vi "Program Set Point.vi"(8 "error in (no error)":errorcluster, 10 "Set Point":dbl, 11 "LakeShore T Controller in":refnum<class "LakeShore T Controller.lvclass">) -> (0 "error out":errorcluster, 3 "LakeShore T Controller out":refnum<class "LakeShore T Controller.lvclass">)   [LabVIEW 2015, in "LakeShore T Controller.lvclass"]
uses:
  LakeShore T Controller.lvclass
  Mag Lab Hardware.lvclass/Mag Lab Hardware.ctl
  Mag Lab Hardware.lvclass
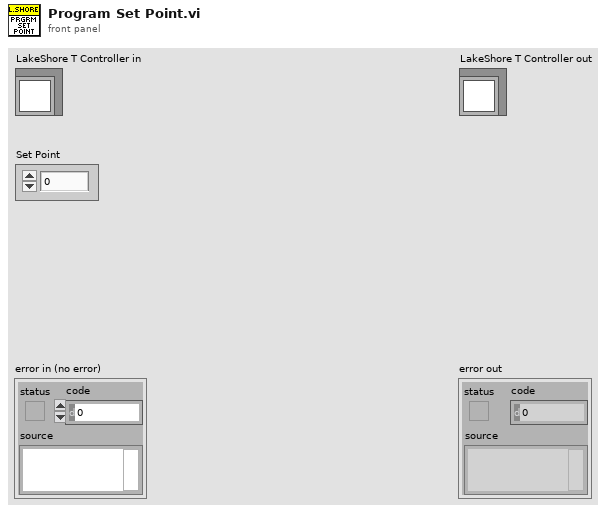
[diagram p1: front panel]
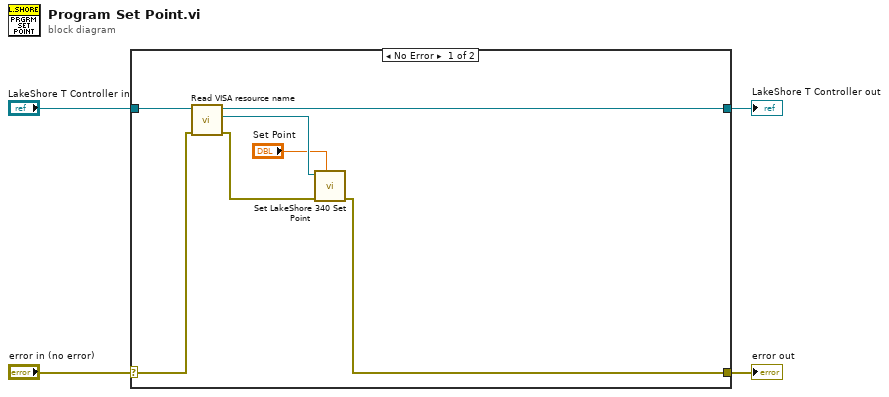
[diagram p0: block diagram]
diagram:
  n1 = case shown="No Error" "error in (no error)" {
    selector: "error in (no error)" -> [w5 w13]
    tunnel: [w7 w13] -> w3
    tunnel: [w10 w12] -> w1
    tunnel: "LakeShore T Controller in" -> [w11 w12]
    frame No Error {
      n2 = call "Read VISA resource name.vi"("error in (no error)"=w5, "Mag Lab Hardware in"=w11) -> ("error out"=w6:errorcluster, "VISA resource name"=w9:refnum<visa-resource-name>, "Mag Lab Hardware out"=w10:refnum<class "LakeShore T Controller.lvclass">)  [unwired: 7 in]
      n3 = call "Set LakeShore 340 Set Point.vi"("Set point"="Set Point", "error in (no error)"=w6, "VISA Resource Name"=w9) -> ("error out"=w7:errorcluster)  [unwired: 7 in, 1 out]
    }
    frame Error {
    }
  }
  "error out" <- w3
  "LakeShore T Controller out" <- w1
